vi "Filter 1D Array__ogtk.vi"   [LabVIEW 2012]
doc: "This polymorphic VI filters out all instances of <B>items to filter</B> from the input <B>array</B> and outputs the result as <B>filtered array</B> along with an array of <B>filtered item indices</B> containing the indices of the items that were filtered. You can wire either a 1D array or a scalar value to <B>items to filter</B>."
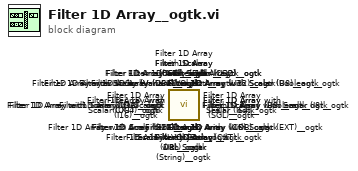
[diagram p0: block diagram]
diagram:
  n1 = call <userlib>:"Filter 1D Array with Scalar (LVObject)__ogtk.vi"() -> ()  [unwired: 6 in, 2 out]
  n2 = call <userlib>:"Filter 1D Array (LVObject)__ogtk.vi"() -> ()  [unwired: 6 in, 2 out]
  n3 = call <userlib>:"Filter 1D Array with Scalar (U64)__ogtk.vi"() -> ()  [unwired: 6 in, 2 out]
  n4 = call <userlib>:"Filter 1D Array with Scalar (I64)__ogtk.vi"() -> ()  [unwired: 6 in, 2 out]
  n5 = call <userlib>:"Filter 1D Array (U64)__ogtk.vi"() -> ()  [unwired: 6 in, 2 out]
  n6 = call <userlib>:"Filter 1D Array (I64)__ogtk.vi"() -> ()  [unwired: 6 in, 2 out]
  n7 = call <userlib>:"Filter 1D Array (I8)__ogtk.vi"() -> ()  [unwired: 6 in, 2 out]
  n8 = call <userlib>:"Filter 1D Array (I16)__ogtk.vi"() -> ()  [unwired: 6 in, 2 out]
  n9 = call <userlib>:"Filter 1D Array (I32)__ogtk.vi"() -> ()  [unwired: 6 in, 2 out]
  n10 = call <userlib>:"Filter 1D Array (U8)__ogtk.vi"() -> ()  [unwired: 6 in, 2 out]
  n11 = call <userlib>:"Filter 1D Array (U16)__ogtk.vi"() -> ()  [unwired: 6 in, 2 out]
  n12 = call <userlib>:"Filter 1D Array (U32)__ogtk.vi"() -> ()  [unwired: 6 in, 2 out]
  n13 = call <userlib>:"Filter 1D Array (Path)__ogtk.vi"() -> ()  [unwired: 6 in, 2 out]
  n14 = call <userlib>:"Filter 1D Array (String)__ogtk.vi"() -> ()  [unwired: 6 in, 2 out]
  n15 = call <userlib>:"Filter 1D Array (Variant)__ogtk.vi"() -> ()  [unwired: 6 in, 2 out]
  n16 = call <userlib>:"Filter 1D Array (Boolean)__ogtk.vi"() -> ()  [unwired: 6 in, 2 out]
  n17 = call <userlib>:"Filter 1D Array (CXT)__ogtk.vi"() -> ()  [unwired: 6 in, 2 out]
  n18 = call <userlib>:"Filter 1D Array (CDB)__ogtk.vi"() -> ()  [unwired: 6 in, 2 out]
  n19 = call <userlib>:"Filter 1D Array (CSG)__ogtk.vi"() -> ()  [unwired: 6 in, 2 out]
  n20 = call <userlib>:"Filter 1D Array (EXT)__ogtk.vi"() -> ()  [unwired: 6 in, 2 out]
  n21 = call <userlib>:"Filter 1D Array (DBL)__ogtk.vi"() -> ()  [unwired: 6 in, 2 out]
  n22 = call <userlib>:"Filter 1D Array (SGL)__ogtk.vi"() -> ()  [unwired: 6 in, 2 out]
  n23 = call <userlib>:"Filter 1D Array with Scalar (Boolean)__ogtk.vi"() -> ()  [unwired: 6 in, 2 out]
  n24 = call <userlib>:"Filter 1D Array with Scalar (CDB)__ogtk.vi"() -> ()  [unwired: 6 in, 2 out]
  n25 = call <userlib>:"Filter 1D Array with Scalar (CSG)__ogtk.vi"() -> ()  [unwired: 6 in, 2 out]
  n26 = call <userlib>:"Filter 1D Array with Scalar (CXT)__ogtk.vi"() -> ()  [unwired: 6 in, 2 out]
  n27 = call <userlib>:"Filter 1D Array with Scalar (DBL)__ogtk.vi"() -> ()  [unwired: 6 in, 2 out]
  n28 = call <userlib>:"Filter 1D Array with Scalar (EXT)__ogtk.vi"() -> ()  [unwired: 6 in, 2 out]
  n29 = call <userlib>:"Filter 1D Array with Scalar (I8)__ogtk.vi"() -> ()  [unwired: 6 in, 2 out]
  n30 = call <userlib>:"Filter 1D Array with Scalar (I16)__ogtk.vi"() -> ()  [unwired: 6 in, 2 out]
  n31 = call <userlib>:"Filter 1D Array with Scalar (I32)__ogtk.vi"() -> ()  [unwired: 6 in, 2 out]
  n32 = call <userlib>:"Filter 1D Array with Scalar (Path)__ogtk.vi"() -> ()  [unwired: 6 in, 2 out]
  n33 = call <userlib>:"Filter 1D Array with Scalar (SGL)__ogtk.vi"() -> ()  [unwired: 6 in, 2 out]
  n34 = call <userlib>:"Filter 1D Array with Scalar (String)__ogtk.vi"() -> ()  [unwired: 6 in, 2 out]
  n35 = call <userlib>:"Filter 1D Array with Scalar (U8)__ogtk.vi"() -> ()  [unwired: 6 in, 2 out]
  n36 = call <userlib>:"Filter 1D Array with Scalar (U16)__ogtk.vi"() -> ()  [unwired: 6 in, 2 out]
  n37 = call <userlib>:"Filter 1D Array with Scalar (U32)__ogtk.vi"() -> ()  [unwired: 6 in, 2 out]
  n38 = call <userlib>:"Filter 1D Array with Scalar (Variant)__ogtk.vi"() -> ()  [unwired: 6 in, 2 out]
